vi "Initialize.vi"(8 "error IO":errorcluster, 10 "Initialization variables":T1={"Channel"=1, "Simulated/Real"=FALSE, "Image path:"=path "E:/images/today", "Remote IP:"="200.131.64.49", "Path to Python.exe"=path "C:/Users/observer/Anaconda3/python.exe", "TCPIP/Stream"=FALSE} {"Channel" min=1 max=4}, 11 "Channel.lvclass":refnum<class "Channel.lvclass">) -> (0 "error IO 2":errorcluster, 2 "Software version":string="v1.14.0", 3 "Channel.lvclass 2":refnum<class "Channel.lvclass">)   [LabVIEW 2018, in "Channel.lvclass"]
doc: "Initialize ACS"
uses:
  Channel.lvclass
  Channel.lvclass/Channel.ctl
  Simulated_CCD_Camera/Simulated_CCD_Camera.lvclass/Simulated_CCD_Camera.ctl
  Simulated_CCD_Camera/Simulated_CCD_Camera.lvclass
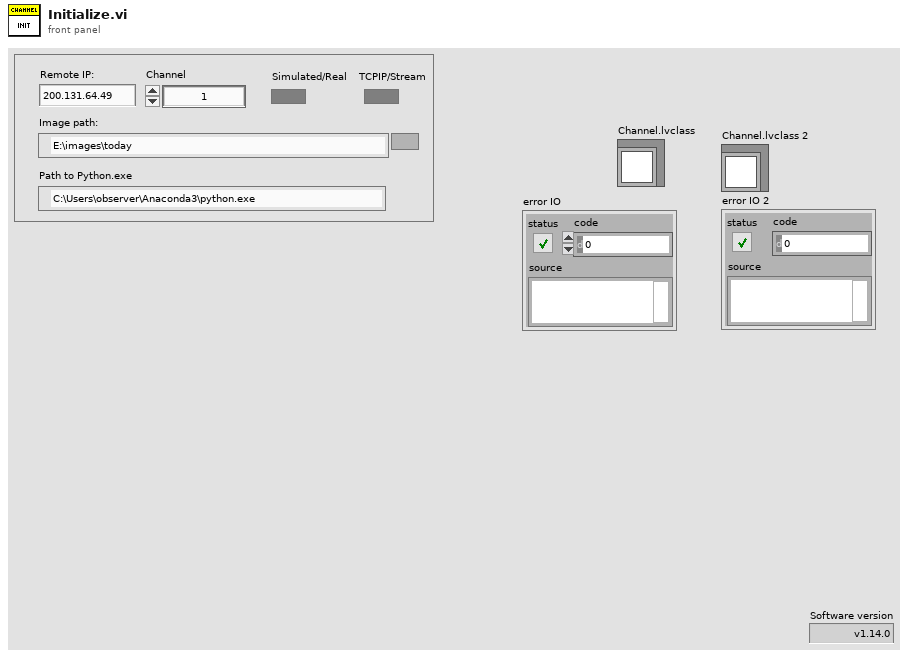
[diagram p1: front panel]
types:
  T1 = cluster{"Channel":u8, "Simulated/Real":bool, "Image path:":path, "Remote IP:":string, "Path to Python.exe":path, "TCPIP/Stream":bool}
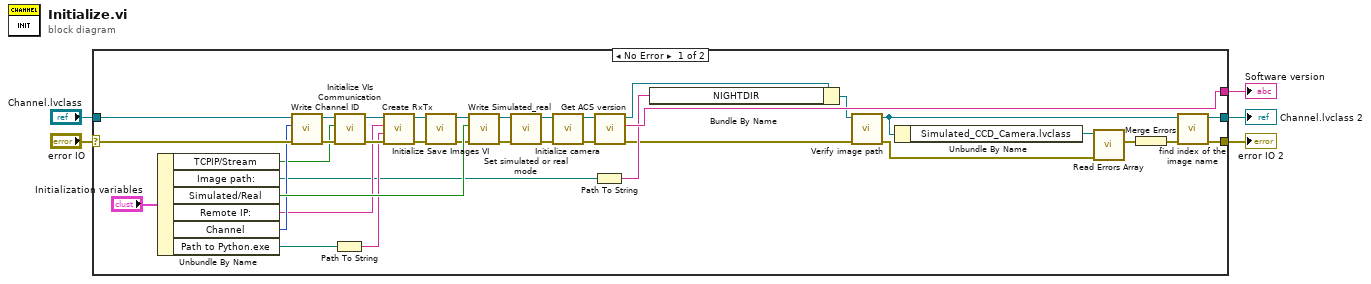
[diagram p0: block diagram]
diagram:
  n1 = case shown="No Error" "error IO" {
    selector: "error IO" -> [w41 w43]
    tunnel: [w17 w43] -> w2
    tunnel: [w18 w42] -> w3
    tunnel: "Channel.lvclass" -> [w33 w42]
    tunnel: [w30 _] -> w1
    frame No Error {
      n2 = Unbundle By Name("Initialization variables") -> ("TCPIP/Stream"=w8:bool, "Image path:"=w20:path, "Simulated/Real"=w36:bool, "Remote IP:"=w31:string, "Channel"=w32:u8, "Path to Python.exe"=w27:path)
      n3 = call "Write Channel ID.vi"("error in (no error)"=w41, "ID"=w32, "Channel in"=w33) -> ("error out"=w24:errorcluster, "Channel out"=w25:refnum<class "Channel.lvclass">)  [unwired: 7 in]
      n4 = Path To String(path=w27) -> (string=w26:string)
      n5 = call "Initialize VIs Communication.vi"("error in (no error)"=w24, "TCPIP/Stream"=w8, "Channel in"=w25) -> ("error out"=w39:errorcluster, "Channel out"=w40:refnum<class "Channel.lvclass">)  [unwired: 7 in]
      n6 = call "Create RxTx.vi"("error in (no error)"=w39, "Python path"=w26, "Remote IP:"=w31, "Channel in"=w40) -> ("error out"=w38:errorcluster, "Channel out"=w37:refnum<class "Channel.lvclass">)  [unwired: 6 in]
      n7 = call "Initialize Save Images VI.vi"("error in (no error)"=w38, "Channel in"=w37) -> ("error out"=w22:errorcluster, "Channel out"=w23:refnum<class "Channel.lvclass">)  [unwired: 8 in]
      n8 = call "Write Simulated_real.vi"("error in (no error)"=w22, "Simulated/real"=w36, "Channel in"=w23) -> ("error out"=w34:errorcluster, "Channel out"=w35:refnum<class "Channel.lvclass">)  [unwired: 7 in]
      n9 = call "Set simulated or real mode.vi"("error in (no error)"=w34, "Channel in"=w35) -> ("error out"=w28:errorcluster, "Channel out"=w29:refnum<class "Channel.lvclass">)  [unwired: 8 in]
      n10 = call "Initialize camera.vi"("error in (no error)"=w28, "Channel in"=w29) -> ("error out"=w15:errorcluster, "Channel out"=w16:refnum<class "Channel.lvclass">)  [unwired: 8 in]
      n11 = Path To String(path=w20) -> (string=w19:string)
      n12 = call "Get ACS version.vi"("error in (no error)"=w15, "Channel in"=w16) -> ("error out"=w14:errorcluster, "ACS version"=w30:string, "Channel out"=w21:refnum<class "Channel.lvclass">)  [unwired: 7 in]
      n13 = Bundle By Name(cluster=w21, "NIGHTDIR"=w19) -> (w13:refnum<class "Channel.lvclass">)
      n14 = call "Verify image path.vi"("error in (no error)"=w14, "Channel in"=w13) -> ("error out"=w11:errorcluster, "Channel out"=w10:refnum<class "Channel.lvclass">)  [unwired: 8 in]
      n15 = Unbundle By Name(w10) -> ("Simulated_CCD_Camera.lvclass"=w12:refnum<class "Simulated_CCD_Camera.lvclass">)
      n16 = call "Read Errors Array.vi"("error in (no error)"=w11, "Simulated_CCD_Camera in"=w12) -> ("Errors array"=w7:errorcluster[])  [unwired: 7 in, 2 out]
      n17 = Merge Errors(w7) -> (w6:errorcluster)
      n18 = call "find index of the image name.vi"("error in (no error)"=w6, "Channel in"=w10) -> ("error out"=w17:errorcluster, "Channel out"=w18:refnum<class "Channel.lvclass">)  [unwired: 8 in]
    }
    frame Error {
    }
  }
  "Channel.lvclass 2" <- w3
  "error IO 2" <- w2
  "Software version" <- w1
